vi "SerialControl.vi"(2 "Set Count":u32=1024, 3 "Input":u8[](array[numeric]), 4 "Mode":u32(ring) items=["Read", "Write", "Query"], 5 "Port":string) -> (0 "Return Count":u32, 1 "Output":u8[](array[numeric]))   [LabVIEW 2011]
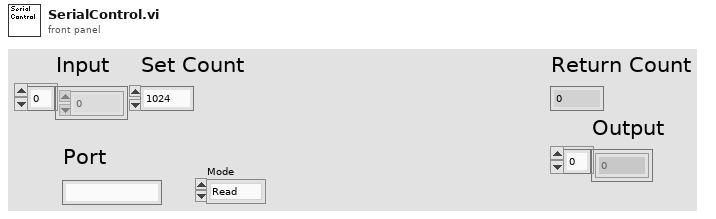
[diagram p1: front panel]
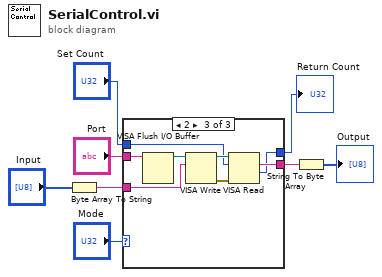
[diagram p0: block diagram]
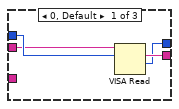
[diagram p2: hidden frame]
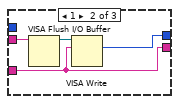
[diagram p3: hidden frame]
diagram:
  n1 = Byte Array To String(unsigned byte array="Input") -> (string=w4:string)
  n2 = case shown="2" "Mode" {
    tunnel: w4 -> [_ w13 w24]
    tunnel: [w12 w13 w22] -> w3
    tunnel: "Set Count" -> [w11 _ w21]
    tunnel: "Port" -> [w10 w16 w19]
    tunnel: [w9 w14 w17] -> w2
    frame 0, Default {
      n3 = VISA Read(VISA resource name=w10, byte count=w11) -> (read buffer=w12:string, return count=w9:u32)  [unwired: 1 in, 2 out]
    }
    frame 1 {
      n4 = VISA Flush I/O Buffer(VISA resource name=w16) -> (VISA resource name out=w15:refnum<visa-resource-name>)  [unwired: 2 in, 1 out]
      n5 = VISA Write(VISA resource name=w15, write buffer=w13) -> (return count=w14:u32)  [unwired: 1 in, 2 out]
    }
    frame 2 {
      n6 = VISA Flush I/O Buffer(VISA resource name=w19) -> (VISA resource name out=w18:refnum<visa-resource-name>)  [unwired: 2 in, 1 out]
      n7 = VISA Write(VISA resource name=w18, write buffer=w24) -> (VISA resource name out=w23:refnum<visa-resource-name>, error out=w20:errorcluster)  [unwired: 1 in, 1 out]
      n8 = VISA Read(VISA resource name=w23, byte count=w21, error in (no error)=w20) -> (read buffer=w22:string, return count=w17:u32)  [unwired: 2 out]
    }
  }
  "Return Count" <- w2
  n9 = String To Byte Array(string=w3) -> (unsigned byte array=→"Output":u8[])
